vi "ASS2-Modulatingsignal.vi"() -> ()   [LabVIEW 2018]
uses:
  <vilib>/measure/NI_MABase.lvlib
panel:
  in  "signal type 2":T1(ring)
  in  "signal type":T1(ring)
  out "Modulated signal":waveform(dbl)(graph)
  out "Carrier signal":waveform(dbl)(graph)
  out "Modulating signal":waveform(dbl)(graph)
  in  "amplitude 2":dbl=1.0 format="%0.2p"
  in  "frequency 2":dbl=10.0 format="%0.2p"
  in  "sampling info":cluster{"Fs":dbl, "#s":dbl}={"Fs"=1000.0, "#s"=1000.0} {"Fs" format="%.2p"}
  in  "amplitude":dbl=1.0 format="%0.2p"
  in  "frequency":dbl=10.0 format="%0.2p"
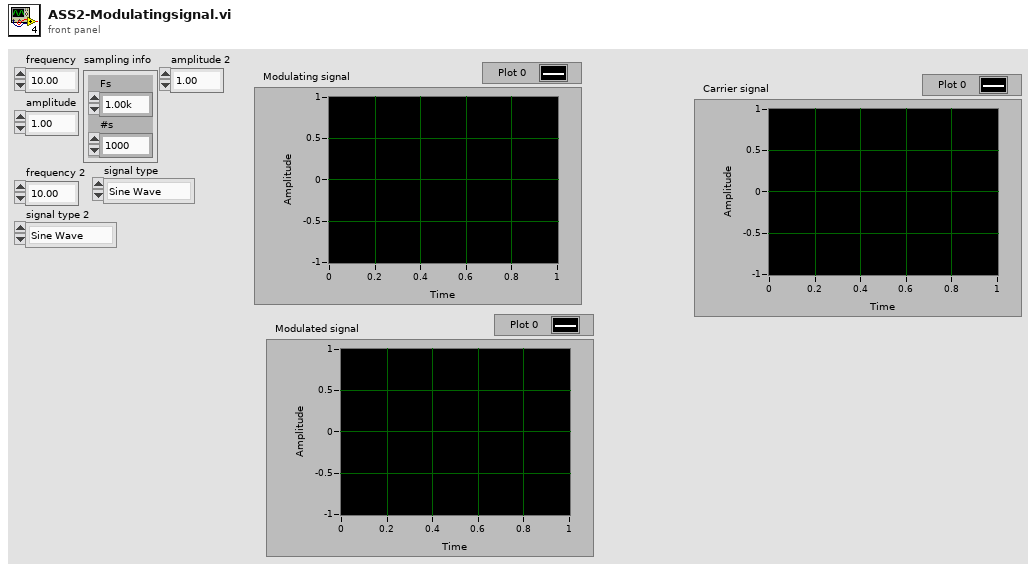
[diagram p1: front panel]
types:
  T1 = enum16{"Sine Wave", "Triangle Wave", "Square Wave", "Sawtooth Wave"}
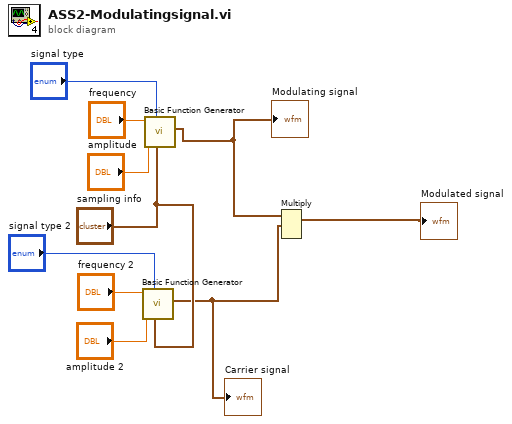
[diagram p0: block diagram]
diagram:
  n1 = call <vilib>:"Basic Function Generator.vi"("sampling info"="sampling info", "signal type"="signal type 2", "amplitude"="amplitude 2", "frequency"="frequency 2") -> ("signal out"=w4:waveform(dbl))  [unwired: 5 in, 2 out]
  "Carrier signal" <- w4
  n2 = call <vilib>:"Basic Function Generator.vi"("sampling info"="sampling info", "signal type"="signal type", "amplitude"="amplitude", "frequency"="frequency") -> ("signal out"=w5:waveform(dbl))  [unwired: 5 in, 2 out]
  "Modulating signal" <- w5
  n3 = Multiply(1:w4, 2:w5) -> (0:→"Modulated signal":waveform(dbl))  [unwired: 1 in, 1 out]
